vi "Update #.vi"(8 "error in (no error)":errorcluster, 11 "Experiments_group in":refnum<class "Experiments_group.lvclass">) -> (0 "error out":errorcluster, 3 "Experiments_group out":refnum<class "Experiments_group.lvclass">)   [LabVIEW 2018, in "Experiments_group.lvclass"]
uses:
  Experiments_group.lvclass
  Experiments_group.lvclass/Experiments_group.ctl
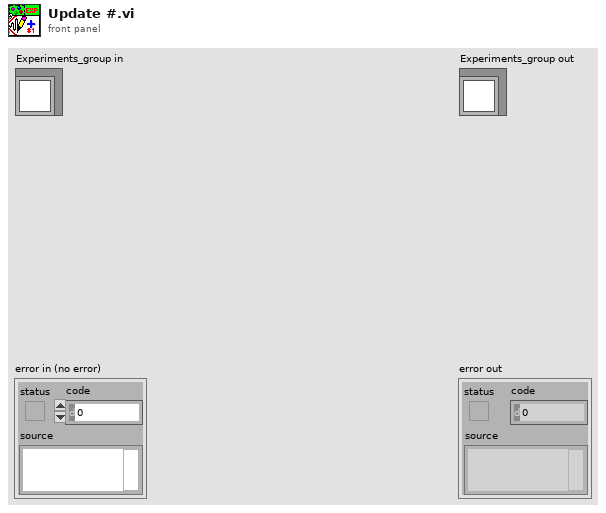
[diagram p1: front panel]
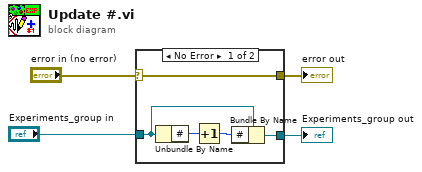
[diagram p0: block diagram]
diagram:
  n1 = case shown="No Error" "error in (no error)" {
    selector: "error in (no error)" -> [w9 w10]
    tunnel: [w9 w10] -> w3
    tunnel: [w8 w11] -> w1
    tunnel: "Experiments_group in" -> [w7 w11]
    frame No Error {
      n2 = Unbundle By Name(w7) -> ("#"=w6:i32)
      n3 = Increment(x=w6) -> (x+1=w5:i32)
      n4 = Bundle By Name(cluster=w7, "#"=w5) -> (w8:refnum<class "Experiments_group.lvclass">)
    }
    frame Error {
    }
  }
  "error out" <- w3
  "Experiments_group out" <- w1
